vi "Multiple VIs in a Subpanel.vi"() -> ()   [LabVIEW 2017, in "MAX_serials.lvclass"]
doc: "This example shows how to view VIs in a Subpanel control."
uses:
  OOD/CLS_MAX_serials/MAX_serials.lvclass
panel:
  in  "VI to Display":u16(ring) items=["Sine Graph", "Random Data Chart", "Current Time"]
  in  "Stop":bool
  # "Overview: Demonstrates the use of the Subpanel control to display different VI panels.\nInstructions:\n1. Run the VI.\n2. Select different options in the VI to Display ring to display different VIs in the subpanel.\n3. Click Stop to stop the VI."
  # "The VI Properties of the inserted VI govern its appearance in the Subpanel control. For example, all of the plugin VIs for this example have their scrollbars disabled. Thus, scrollbars do not appear within the Subpanel control."
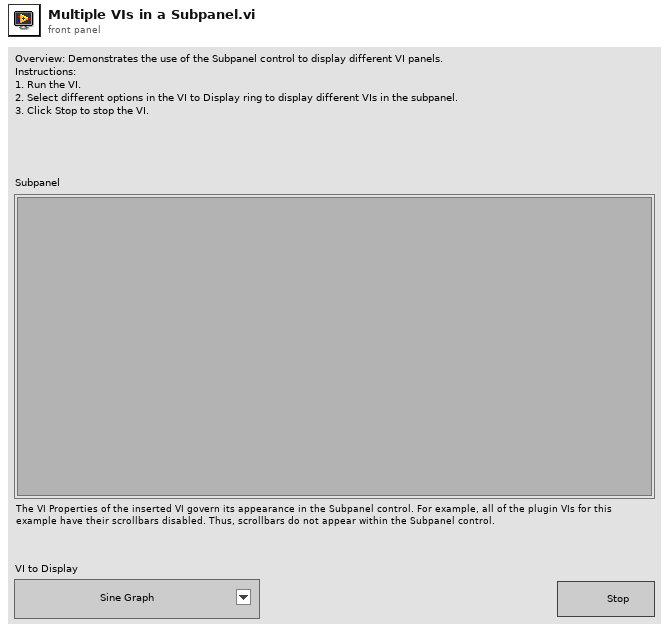
[diagram p1: front panel]
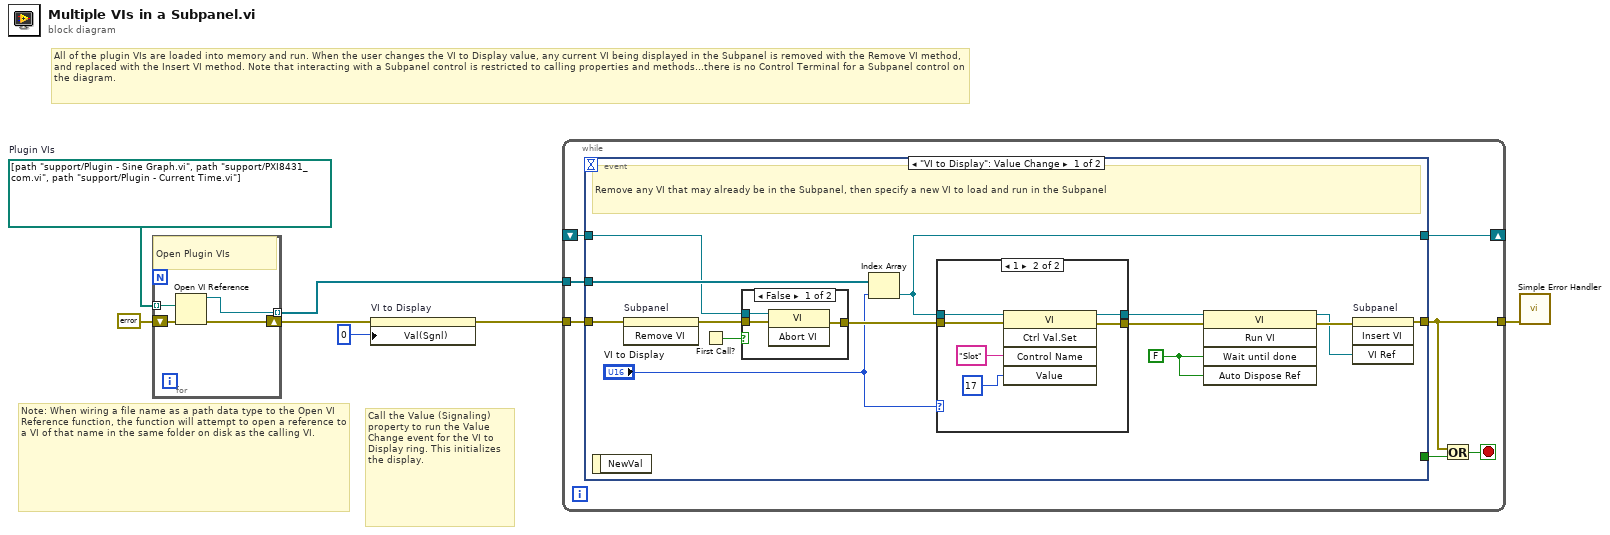
[diagram p0: block diagram]
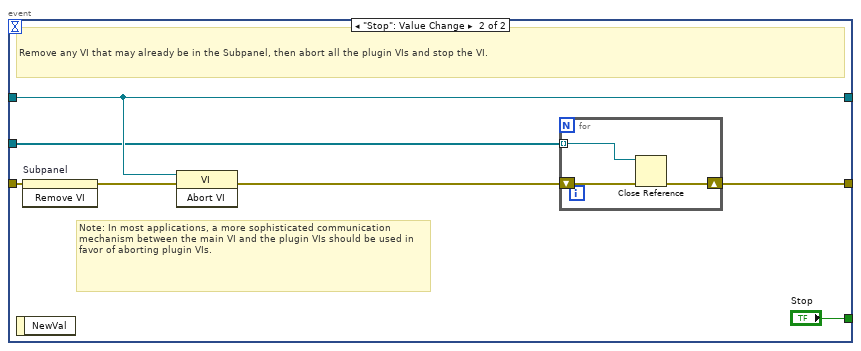
[diagram p4: hidden frame]
diagram:
  w4 = path[] [path "support/Plugin - Sine Graph.vi", path "support/PXI8431_com.vi", path "support/Plugin - Current Time.vi"]  # Plugin VIs
  # "All of the plugin VIs are loaded into memory and run. When the user changes the VI to Display value, any current VI being displayed in the Subpanel is removed with the Remove VI method, and replaced with the Insert VI method. Note that interacting with a Subpanel control is restricted to calling properties and methods...there is no Control Terminal for a Subpanel control on the diagram."
  # "Note: When wiring a file name as a path data type to the Open VI Reference function, the function will attempt to open a reference to a VI of that name in the same folder on disk as the calling VI."
  # "Call the Value (Signaling) property to run the Value Change event for the VI to Display ring. This initializes the display."
  n1 = for {
    tunnel: w4 -> [w11] mode=indexing
    tunnel: [w8] -> w1 mode=indexing
    shift-right: [w9] -> w2
    shift-left: errorcluster {"status"=FALSE, "code"=0, "source"=""} ("error constant") -> [w10]
    # "Open Plugin VIs"
    n2 = Open VI Reference(vi path=w11, error in (no error)=w10) -> (vi reference=w8:refnum<vi>, error out=w9:errorcluster)  [unwired: 4 in]
  }
  n3 = property on="VI to Display" class="Ring (strict)"(error in=w2, "Val(Sgnl)"=u16 0 ("Value (Signaling)")) -> (error out=w7:errorcluster)  [unwired: 1 in, 1 out]
  n4 = while {
    tunnel: w7 -> [w14]
    tunnel: [w16] -> w5
    tunnel: w1 -> [w15]
    shift-right: [w13] -> _
    shift-left: _ -> [w12]
    stop <- w17 stop-if-true
    n5 = event shown="[0] \"VI to Display\": Value Change" {
      selector: _ -> [_ _]
      dyn-events: _ -> [_ _]
      timeout: _ -> [_ _]
      tunnel: [_ "Stop"] -> w18
      tunnel: [w32 w49] -> w16
      tunnel: w15 -> [w31 w45]
      tunnel: w14 -> [w30 w48]
      tunnel: [w27 w46] -> w13
      tunnel: w12 -> [w28 w46]
      event "VI to Display": Value Change {
        w26 = FALSE
        # "Remove any VI that may already be in the Subpanel, then specify a new VI to load and run in the Subpanel"
        n6 = event-data() -> ()  [unwired: 1 in, 1 out]
        n7 = invoke on="Subpanel" class="SubPnl" method="Remove VI"(error in=w30) -> (error out=w29:errorcluster)  [unwired: 2 in, 2 out]
        n8 = First Call?() -> (First Call?: T/F=w23:bool)
        n9 = case shown="False" w23 {
          tunnel: w29 -> [w43 w44]
          tunnel: w28 -> [w42 _]
          tunnel: [w41 w44] -> w21
          frame False {
            n10 = invoke class="VI" method="Abort VI"(reference=w42, error in=w43) -> (error out=w41:errorcluster)  [unwired: 1 in, 2 out]
          }
          frame True {
          }
        }
        n11 = Index Array(array=w31, index="VI to Display") -> (element=w27:refnum<vi>)
        n12 = case shown="1" "VI to Display" {
          tunnel: w27 -> [w34 w40]
          tunnel: [w34 w39] -> w22
          tunnel: w21 -> [w33 w38]
          tunnel: [w33 w37] -> w20
          frame 0, Default {
          }
          frame 1 {
            n13 = invoke class="VI" method="Ctrl Val.Set"(reference=w40, error in=w38, "Control Name"="Slot", "Value"=17) -> (reference out=w39:refnum<vi>, error out=w37:errorcluster)  [unwired: 1 in, 3 out]
          }
        }
        n14 = invoke class="VI" method="Run VI"(reference=w22, error in=w20, "Wait until done"=w26, "Auto Dispose Ref"=w26) -> (reference out=w24:refnum<vi>, error out=w25:errorcluster)  [unwired: 1 in, 3 out]
        n15 = invoke on="Subpanel" class="SubPanel" method="Insert VI"(error in=w25, "VI Ref"=w24) -> (error out=w32:errorcluster)  [unwired: 2 in, 3 out]
      }
      event "Stop": Value Change {
        # "Note: In most applications, a more sophisticated communication mechanism between the main VI and the plugin VIs should be used in favor of aborting plugin VIs."
        # "Remove any VI that may already be in the Subpanel, then abort all the plugin VIs and stop the VI."
        n16 = event-data() -> ()  [unwired: 1 in, 1 out]
        n17 = invoke on="Subpanel" class="SubPnl" method="Remove VI"(error in=w48) -> (error out=w50:errorcluster)  [unwired: 2 in, 2 out]
        n18 = invoke class="VI" method="Abort VI"(reference=w46, error in=w50) -> (error out=w47:errorcluster)  [unwired: 1 in, 2 out]
        n19 = for {
          shift-right: [w54] -> w49
          shift-left: w47 -> [w53]
          tunnel: w45 -> [w52] mode=indexing
          n20 = Close Reference(reference=w52, error in (no error)=w53) -> (error out=w54:errorcluster)
        }
      }
    }
    n21 = Or(x=w16, y=w18) -> (x .or. y?=w17:bool)
  }
  n22 = call <vilib>:"Simple Error Handler.vi"("error in (no error)"=w5) -> ()  [unwired: 4 in, 5 out]
